vi "GT Pt Space.vi"(7 "fifo":i16, 8 "error in (no error)":errorcluster caption="错误输入（无错误）", 9 "pSpace":i16, 10 "profile":i16, 11 "cardNum":i16) -> (0 "error out":errorcluster caption="错误输出", 1 "pSpace out":i16, 3 "function return":i16)   [LabVIEW 2014, in "gts.lvlib"]
doc: "GT_API GT_PtSpace(short cardNum,short profile,short *pSpace,short fifo=0);"
uses:
  gts.lvlib
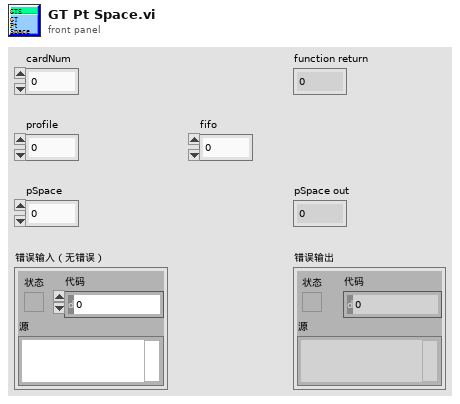
[diagram p1: front panel]
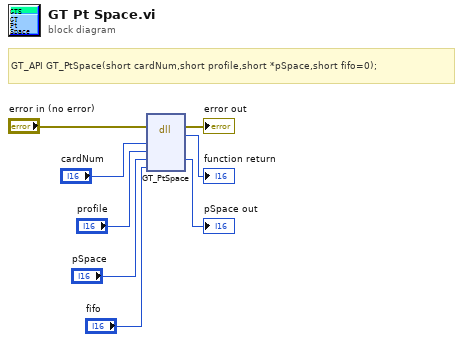
[diagram p0: block diagram]
diagram:
  # "GT_API GT_PtSpace(short cardNum,short profile,short *pSpace,short fifo=0);"
  n1 = dll-call lib="PTH2habs D固高科技资料GTS控制卡GTS卡18年上半年资料dllVC32bit\nmulti_cardgts.*" fn="GT_PtSpace"(error in="error in (no error)", "cardNum"="cardNum", "profile"="profile", "pSpace"="pSpace", "fifo"="fifo") -> (error out=→"error out":errorcluster, →"function return":i16, "pSpace"=→"pSpace out":i16)  [unwired: 5 in, 1 out]
